vi "Setup Dialog.vi"() -> ()   [LabVIEW 2011, in "CAN FD.lvlib"]
uses:
  CAN FD.lvlib
  Typedef/Config.ctl
panel:
  in  "OK":bool
  in  "ListLen":u32=1000 caption="缓存帧数" min=1000 max=10000000
  in  "Data Format":u16(ring) caption="数据格式" items=["十六进制", "十进制", "二进制", "ASCII码"]
  in  "ID Format":u16(ring) caption="ID格式" items=["十六进制", "十进制"]
  in  "TimeFormat":u16(ring) caption="时间格式" items=["系统时间", "时间戳(s)"]
  # "设置参数"
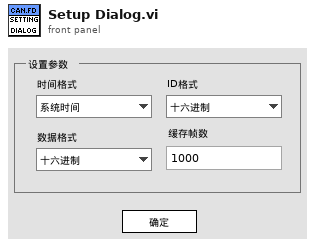
[diagram p1: front panel]
types:
  T1 = typedef "CAN FD.lvlib/Config.ctl" = cluster{"TimeFormat":u16, "ID Format":u16, "Data Format":u16, "ListLen":u32}
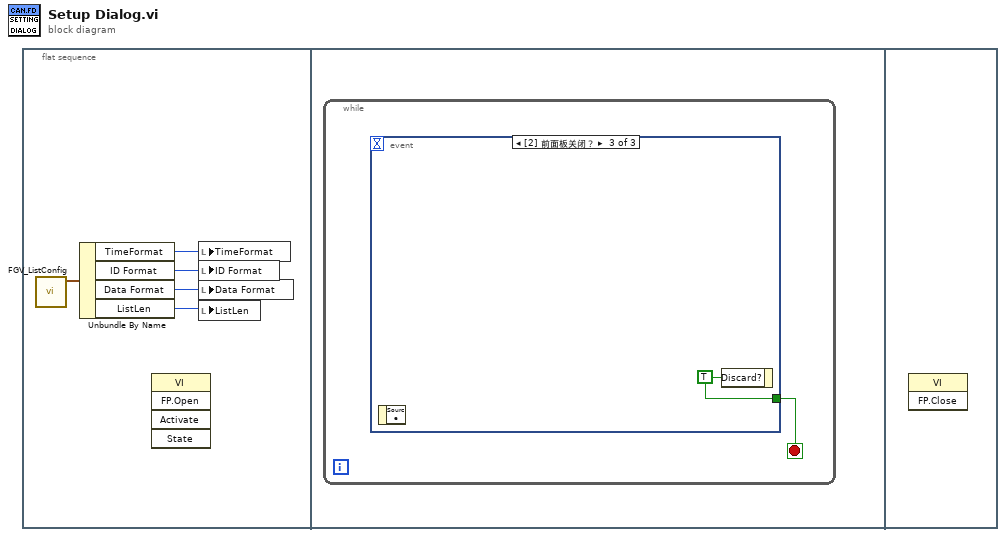
[diagram p0: block diagram]
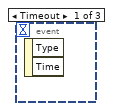
[diagram p2: hidden frame]
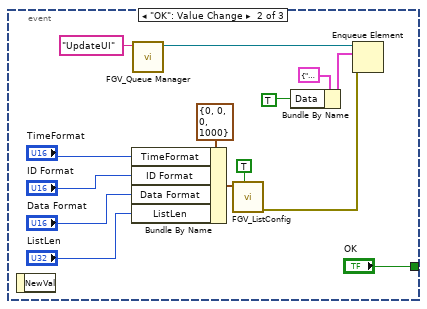
[diagram p3: hidden frame]
diagram:
  n1 = flat-sequence {
    frame #0 {
      n2 = call "FGV_ListConfig.vi"() -> ("Config out"=w1:T1)  [unwired: 10 in, 1 out]
      n3 = Unbundle By Name(w1) -> ("TimeFormat"=w2:u16, "ID Format"=w4:u16, "Data Format"=w3:u16, "ListLen"=w5:u32)
      n4 = invoke class="VI" method="FP.Open"() -> ()  [unwired: 5 in, 5 out]
      n5 = local write "TimeFormat"(w2) -> ()
      n6 = local write "ID Format"(w4) -> ()
      n7 = local write "Data Format"(w3) -> ()
      n8 = local write "ListLen"(w5) -> ()
    }
    frame #1 {
      n9 = while {
        stop <- w6 stop-if-true
        n10 = event shown="[2] 前面板关闭？" {
          selector: _ -> [_ _ _]
          dyn-events: _ -> [_ _ _]
          timeout: _ -> [_ _ _]
          tunnel: [_ "OK" w21] -> w6
          event Timeout {
            n11 = event-data() -> ()  [unwired: 1 in, 2 out]
          }
          event "OK": Value Change {
            n12 = event-data() -> ()  [unwired: 1 in, 1 out]
            n13 = Bundle By Name(cluster=T1 {"TimeFormat"=0, "ID Format"=0, "Data Format"=0, "ListLen"=1000} ("Config"), "TimeFormat"="TimeFormat", "ID Format"="ID Format", "Data Format"="Data Format", "ListLen"="ListLen") -> (w15:T1)
            n14 = call "FGV_Queue Manager.vi"("Name"="UpdateUI") -> ("Queue"=w8:refnum<queue>)  [unwired: 8 in, 2 out]
            n15 = call "FGV_ListConfig.vi"("Set"=TRUE, "Config"=w15) -> ("error out"=w7:errorcluster)  [unwired: 8 in, 1 out]
            n16 = Bundle By Name(cluster=cluster{"ID":string, "Data":variant} {"ID"="Update", "Data"=variant} ("元素"), "Data"=TRUE) -> (w9:cluster{"ID":string, "Data":variant})
            n17 = Enqueue Element(queue=w8, element=w9, error in (no error)=w7) -> ()  [unwired: 1 in, 3 out]
          }
          event Panel Close? {
            w21 = TRUE ("放弃？")
            n18 = event-data() -> ()  [unwired: 1 in, 1 out]
            n19 = event-data("Discard?"=w21) -> ()  [unwired: 1 in, 1 out]
          }
        }
      }
    }
    frame #2 {
      n20 = invoke class="VI" method="FP.Close"() -> ()  [unwired: 3 in, 3 out]
    }
  }
